vi "GDSLvIcon_AnalyseViIcon.vi"(1 "ViRef/LvCLassRef/LvLibRef/ViPath/2D_Image":variant, 3 "DoATextOCR(False)":bool, 5 "error in (no error)":errorcluster) -> (6 "BodyTextColor":u32(colorbox), 8 "HeaderTextColor":u32(colorbox), 9 "BodyText(OCR)":string, 10 "FrameColor":u32(colorbox), 11 "HeadText(OCR)":string, 12 "FrameThickness(1)":u32=1, 13 "ValidHeaderIcon":bool, 14 "DefaultIcon":bool, 15 "HeaderIcon":u8[][](array[numeric]) format="%x", 16 "HeaderBkColor":u32(colorbox), 17 "BodyIcon":u8[][](array[numeric]) format="%x", 18 "BodyBkColor":u32(colorbox), 19 "error out":errorcluster)   [LabVIEW 2014]
uses:
  <vilib>/picture/picture.llb/imagedata.ctl
  <vilib>/Analysis/NI_AALBase.lvlib
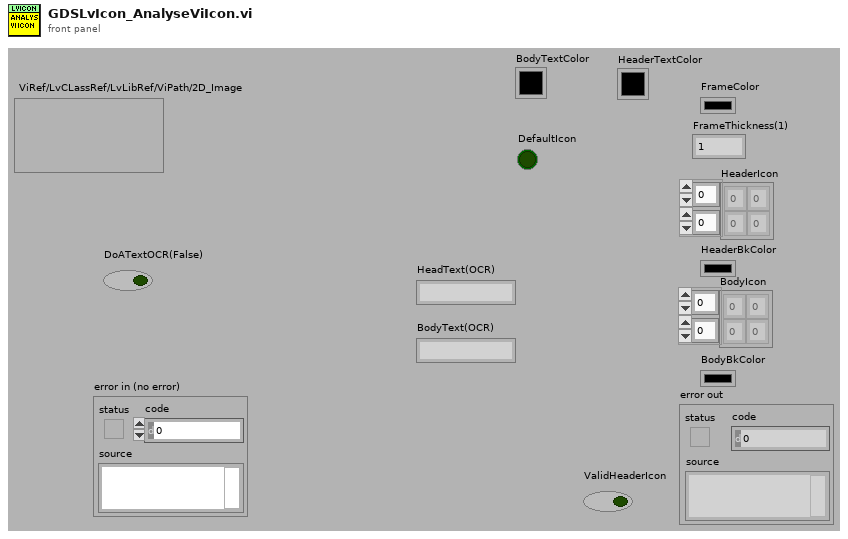
[diagram p1: front panel]
types:
  T1 = cluster{"image":u8[][], "FrameThickness":i32, "FrameColor":u32, "HeaderBkColor":u32, "BodyBkColor":u32, "SplitterAtRow":i32, "Header":u8[][], "Body":u8[][], "HeadTextColor":u32, "BodyTextColor":u32, "BodyBack(8bit)":u8, "BodyText(OCR)":string, "HeadText(OCR)":string, "HeaderBack(8bit)":u8, "EndRow":i32, "StartRow":i32, "BodyTextColor(8bit)":u8, "HeaderTextColor(8bit)":u8, "ShouldHaveHeader":bool}
  T2 = typedef "imagedata.ctl" = cluster{"image type":i32, "image depth":i32, "image":u8[], "mask":u8[], "colors":u32[], "Rectangle":cluster{"left":i16, "top":i16, "right":i16, "bottom":i16}}
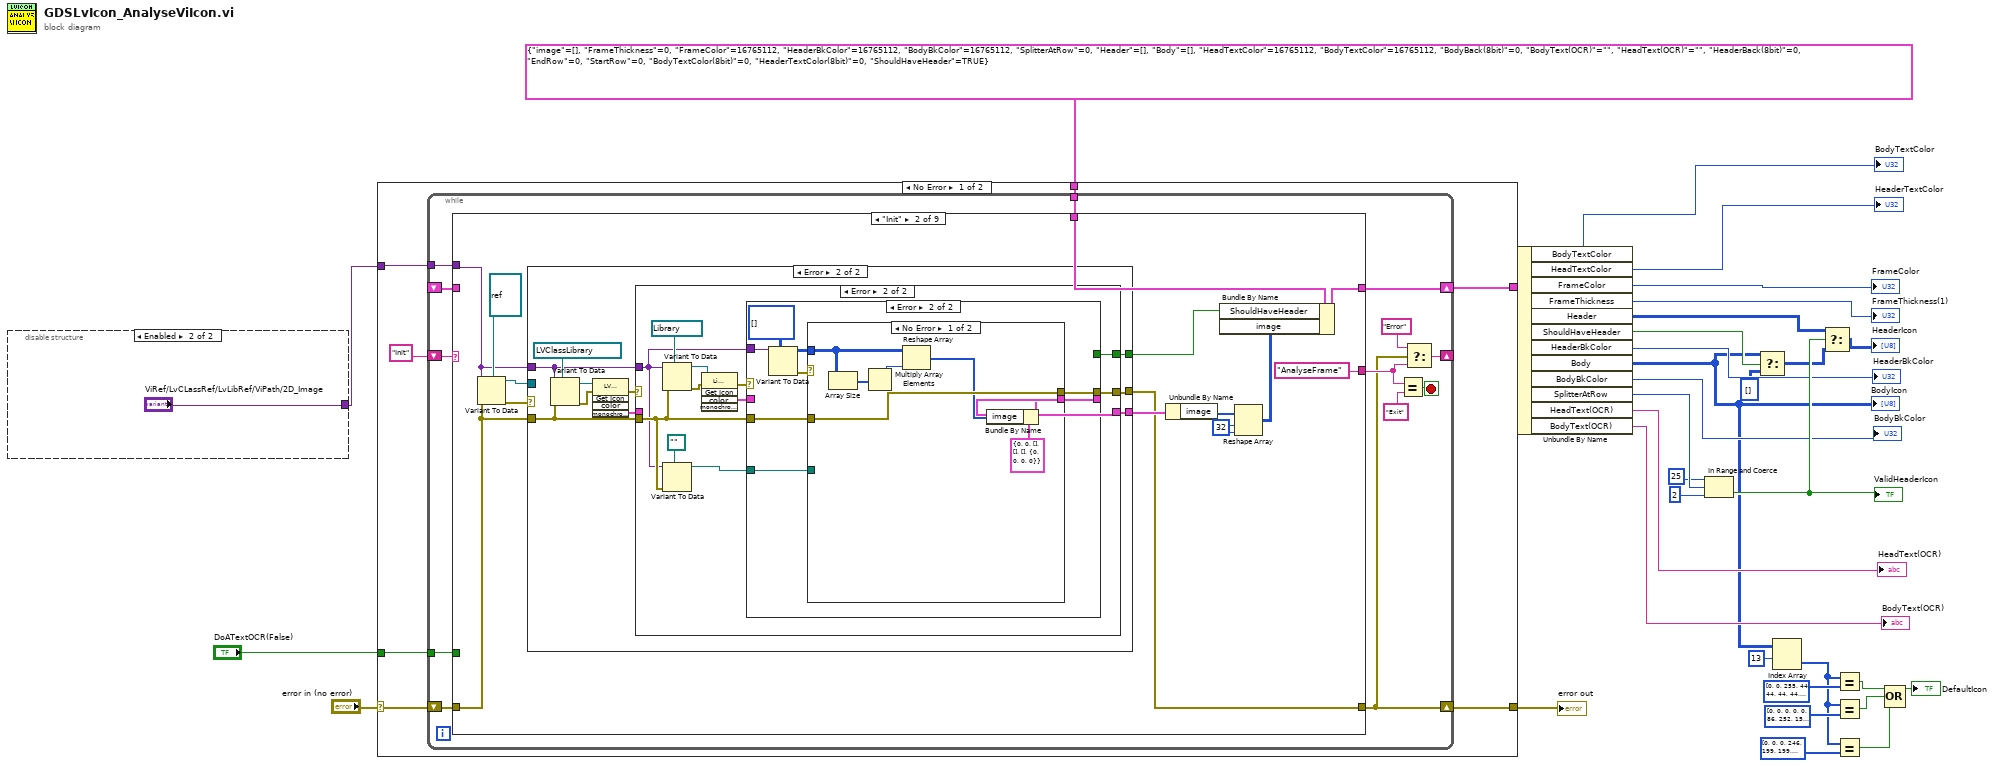
[diagram p0: block diagram]
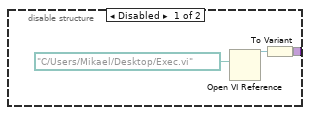
[diagram p2: hidden frame]
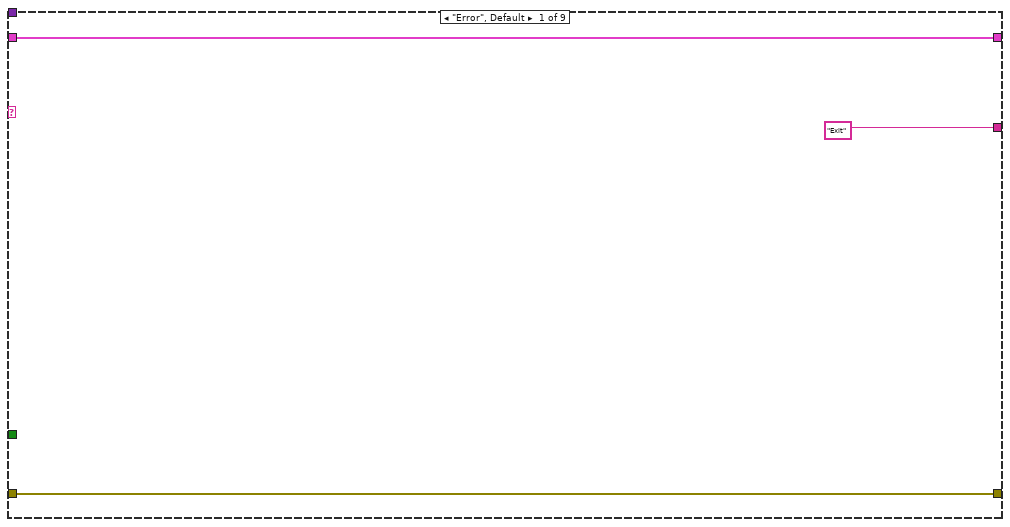
[diagram p3: hidden frame]
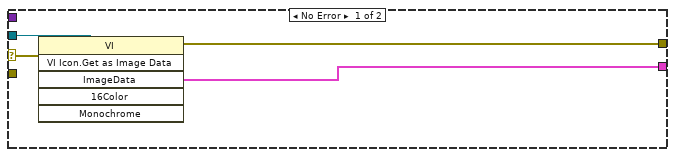
[diagram p4: hidden frame]
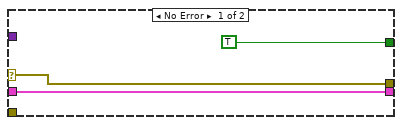
[diagram p6: hidden frame]
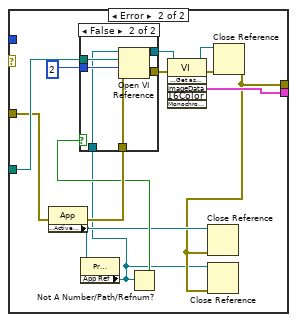
[diagram p7: hidden frame]
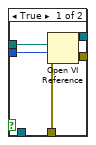
[diagram p8: hidden frame]
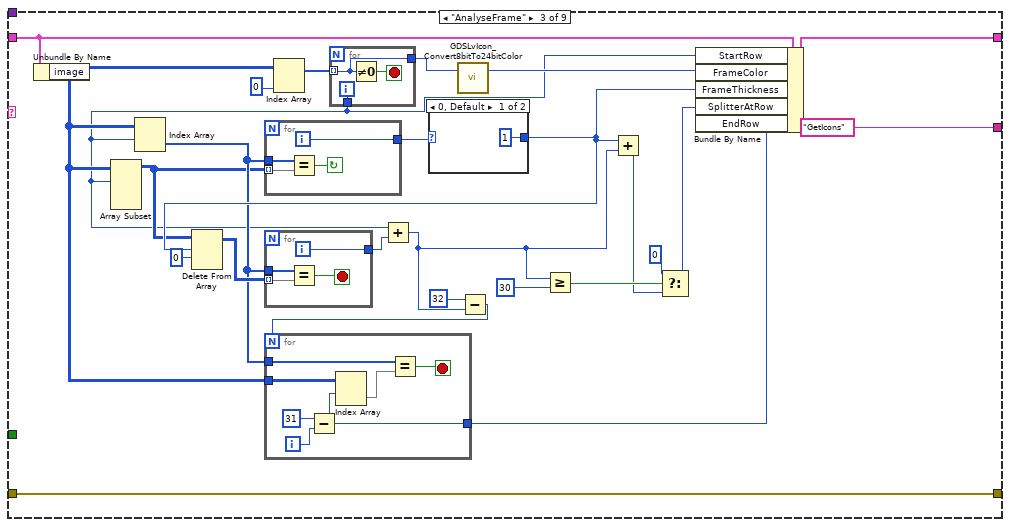
[diagram p9: hidden frame]
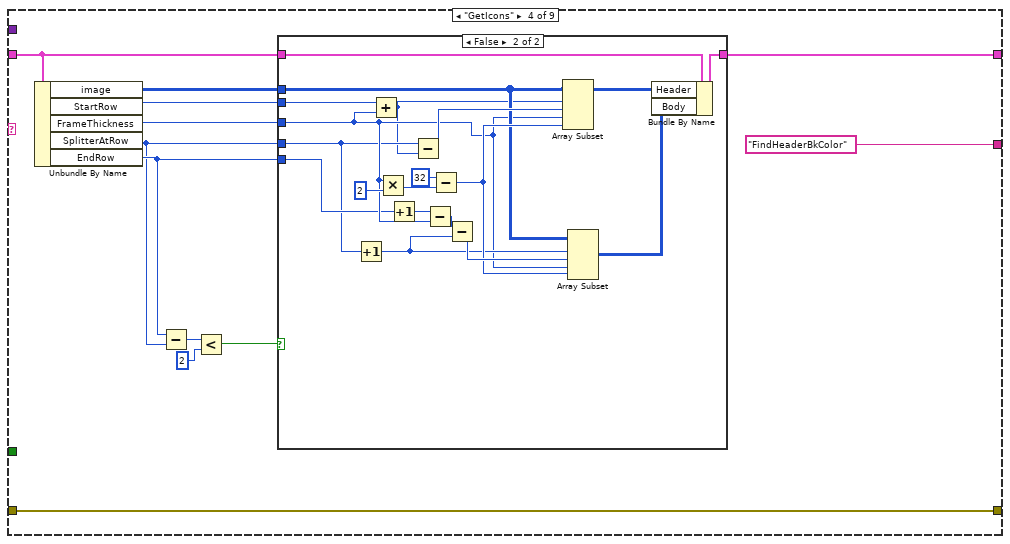
[diagram p11: hidden frame]
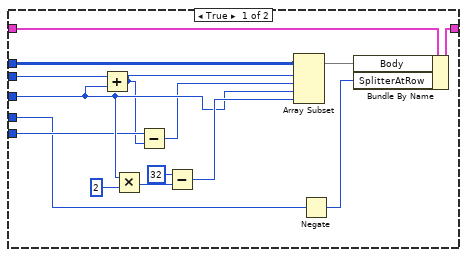
[diagram p12: hidden frame]
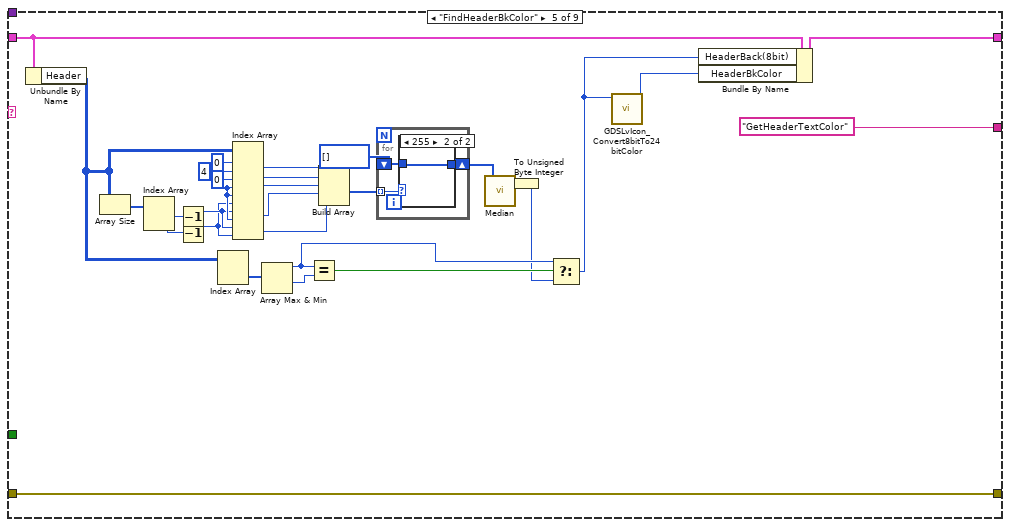
[diagram p13: hidden frame]
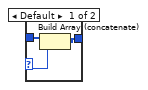
[diagram p14: hidden frame]
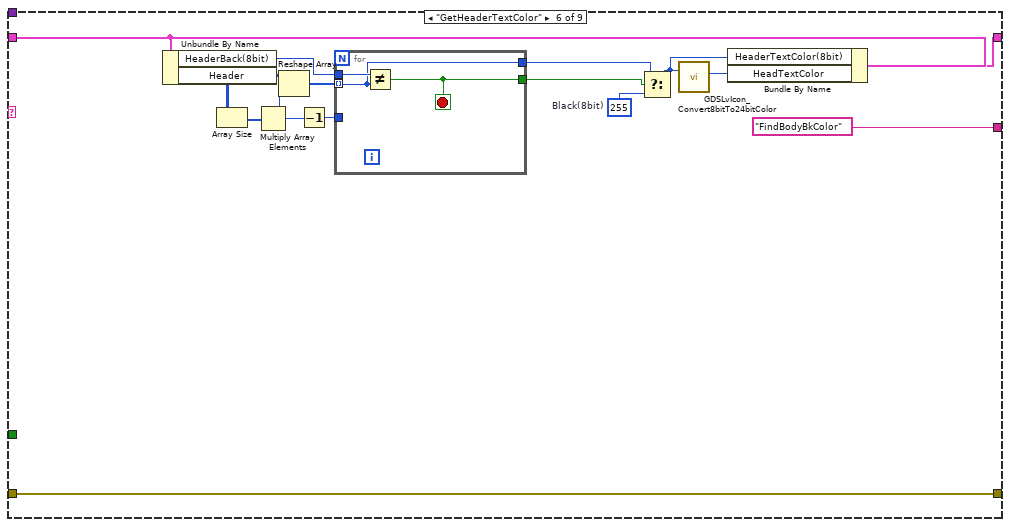
[diagram p15: hidden frame]
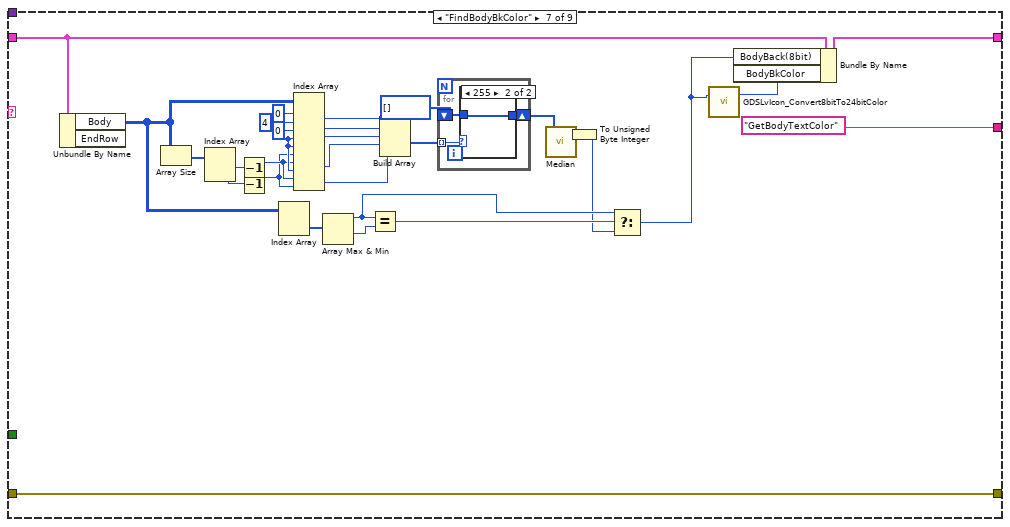
[diagram p16: hidden frame]
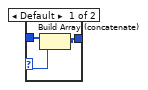
[diagram p17: hidden frame]
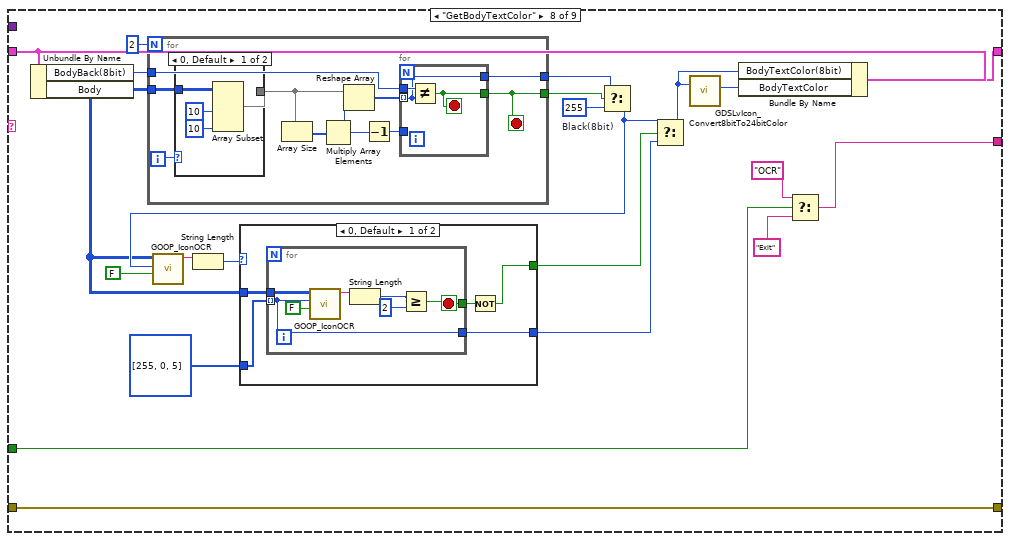
[diagram p18: hidden frame]
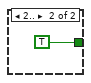
[diagram p19: hidden frame]
diagram:
  n1 = disable-structure shown="Enabled" {
    disable-tunnel: [w34 "ViRef/LvCLassRef/LvLibRef/ViPath/2D_Image"] -> w14
    frame Disabled {
      n2 = Open VI Reference(vi path=path "C:/Users/Mikael/Desktop/Exec.vi") -> (vi reference=w36:refnum<vi>)  [unwired: 5 in, 1 out]
      n3 = To Variant(anything=w36) -> (Variant=w34:variant)
    }
    frame Enabled {
    }
  }
  n4 = case shown="No Error" "error in (no error)" {
    selector: "error in (no error)" -> [w43 w405]
    tunnel: w14 -> [w41 _]
    tunnel: [w42 w405] -> w32
    tunnel: [w40 _] -> w31
    tunnel: T1 {"image"=[], "FrameThickness"=0, "FrameColor"=16765112, "HeaderBkColor"=16765112, "BodyBkColor"=16765112, "SplitterAtRow"=0, "Header"=[], "Body"=[], "HeadTextColor"=16765112, "BodyTextColor"=16765112, "BodyBack(8bit)"=0, "BodyText(OCR)"="", "HeadText(OCR)"="", "HeaderBack(8bit)"=0, "EndRow"=0, "StartRow"=0, "BodyTextColor(8bit)"=0, "HeaderTextColor(8bit)"=0, "ShouldHaveHeader"=TRUE} -> [w39 _]
    tunnel: "DoATextOCR(False)" -> [w38 _]
    frame No Error {
      n5 = while {
        shift-right: [w50] -> w42
        shift-left: w43 -> [w57]
        shift-right: [w55] -> _
        shift-left: "Init" -> [w56]
        shift-right: [w49] -> w40
        shift-left: _ -> [w48]
        tunnel: w41 -> [w47]
        tunnel: w39 -> [w46]
        tunnel: w38 -> [w45]
        stop <- w54 stop-if-true
        n6 = case shown="\"Init\"" w56 {
          tunnel: w57 -> [w60 w64 w165 w199 w264 w286 w319 w348 w389]
          tunnel: [w60 w63 w165 w199 w264 w286 w319 w348 w389] -> w50
          tunnel: ["Exit" "AnalyseFrame" "GetIcons" "FindHeaderBkColor" "GetHeaderTextColor" "FindBodyBkColor" "GetBodyTextColor" w339 "Exit"] -> w51
          tunnel: [w58 w72 w169 w201 w262 w284 w317 w346 w394] -> w49
          tunnel: w48 -> [w58 _ w170 w202 w263 w285 w318 w347 w392]
          tunnel: w47 -> [_ w67 _ _ _ _ _ _ _]
          tunnel: w46 -> [_ w70 _ _ _ _ _ _ _]
          tunnel: w45 -> [_ _ _ _ _ _ _ w341 _]
          frame "Error", Default {
          }
          frame "Init" {
            w61 = 32 ("dimension size")
            n7 = Variant To Data(error in=w64, type=refnum<vi> refnum ("ViRef or LvCLassRef"), Variant=w67) -> (data=w66:refnum<vi>, error out=w68:errorcluster)
            n8 = case shown="Error" w68 {
              selector: w68 -> [w77 _]
              tunnel: w67 -> [_ w81]
              tunnel: w66 -> [w78 _]
              tunnel: [w76 w82] -> w65
              tunnel: w64 -> [_ w80]
              tunnel: [w75 w84] -> w63
              tunnel: [_ w79] -> w62
              frame No Error {
                n9 = invoke class="VI" method="VI Icon.Get as Image Data"(reference=w78, error in=w77) -> (error out=w75:errorcluster, "ImageData"=w76:T2)  [unwired: 4 in, 4 out]
              }
              frame Error {
                n10 = Variant To Data(error in=w80, type=refnum<vi> refnum ("LVClassLibrary Refnum"), Variant=w81) -> (data=w87:refnum<vi>, error out=w86:errorcluster)
                n11 = invoke class="LVClassLibrary" method="Get Icon"(reference=w87, error in=w86) -> (error out=w85:errorcluster, "color"=w83:T2)  [unwired: 3 in, 3 out]
                n12 = case shown="Error" w85 {
                  selector: w85 -> [w90 _]
                  tunnel: [w90 w96] -> w84
                  tunnel: w83 -> [w89 _]
                  tunnel: [w89 w97] -> w82
                  tunnel: w81 -> [_ w91]
                  tunnel: w80 -> [_ w93]
                  tunnel: [_ w92] -> w79
                  frame No Error {
                  }
                  frame Error {
                    n13 = Variant To Data(error in=w93, type=refnum<vi> refnum ("Library Refnum"), Variant=w91) -> (data=w101:refnum<vi>, error out=w100:errorcluster)
                    n14 = Variant To Data(error in=w93, type=path "", Variant=w91) -> (data=w94:path)  [unwired: 1 out]
                    n15 = invoke class="Library" method="Get Icon"(reference=w101, error in=w100) -> (error out=w99:errorcluster, "color"=w98:T2)  [unwired: 3 in, 3 out]
                    n16 = case shown="Error" w99 {
                      selector: w99 -> [w104 _]
                      tunnel: w98 -> [w105 _]
                      tunnel: [w105 w112] -> w97
                      tunnel: [w104 w110] -> w96
                      tunnel: w94 -> [_ w113]
                      tunnel: w93 -> [_ w111]
                      tunnel: [TRUE _] -> w92
                      tunnel: w91 -> [_ w109]
                      frame No Error {
                      }
                      frame Error {
                        n17 = Variant To Data(type=u8[][] [] ("output array"), Variant=w109) -> (data=w106:u8[][], error out=w107:errorcluster)  [unwired: 1 in]
                        n18 = case shown="No Error" w107 {
                          tunnel: w113 -> [_ w133]
                          tunnel: [w118 w128] -> w112
                          tunnel: w111 -> [w120 w126]
                          tunnel: [w120 w122] -> w110
                          tunnel: w106 -> [w117 _]
                          frame No Error {
                            n19 = Array Size(array=w117) -> (size(s)=w115:i32[])
                            n20 = Multiply Array Elements(1:w115) -> (0:w116:i32)
                            n21 = Reshape Array(w117, w116) -> (w114:u8[])
                            n22 = Bundle By Name(cluster=T2 {"image type"=0, "image depth"=0, "image"=[], "mask"=[], "colors"=[], "Rectangle"={"left"=0, "top"=0, "right"=0, "bottom"=0}} ("ImageData"), "image"=w114) -> (w118:T2)
                          }
                          frame Error {
                            n23 = property class="App"(error in=w126) -> (error out=w125:errorcluster, "Project:Active Project"=w123:refnum<vi>)  [unwired: 1 in, 1 out]
                            n24 = property class="Project"(reference=w123) -> ("App Ref"=w121:refnum<vi>)  [unwired: 1 in, 2 out]
                            n25 = Not A Number/Path/Refnum?(number/path/refnum=w121) -> (NaN/Path/Refnum?=w124:bool)
                            n26 = case shown="False" w124 {
                              tunnel: w133 -> [w138 w144]
                              tunnel: [w137 w143] -> w132
                              tunnel: [w136 w142] -> w131
                              tunnel: 2 ("options") -> [w135 w141]
                              tunnel: w125 -> [w134 w140]
                              tunnel: w121 -> [_ w139]
                              frame True {
                                n27 = Open VI Reference(vi path=w138, options=w135, error in (no error)=w134) -> (vi reference=w136:refnum<vi>, error out=w137:errorcluster)  [unwired: 3 in]
                              }
                              frame False {
                                n28 = Open VI Reference(application reference (local)=w139, vi path=w144, options=w141, error in (no error)=w140) -> (vi reference=w142:refnum<vi>, error out=w143:errorcluster)  [unwired: 2 in]
                              }
                            }
                            n29 = invoke class="VI" method="VI Icon.Get as Image Data"(reference=w131, error in=w132) -> (reference out=w129:refnum<vi>, error out=w130:errorcluster, "ImageData"=w128:T2)  [unwired: 4 in, 3 out]
                            n30 = Close Reference(reference=w129, error in (no error)=w130) -> (error out=w122:errorcluster)
                            n31 = Close Reference(reference=w123, error in (no error)=w122) -> ()  [unwired: 1 out]
                            n32 = Close Reference(reference=w121, error in (no error)=w122) -> ()  [unwired: 1 out]
                          }
                        }
                      }
                    }
                  }
                }
              }
            }
            n33 = Unbundle By Name(w65) -> ("image"=w73:u8[])
            n34 = Reshape Array(w73, w61, w61) -> (w71:u8[][])
            n35 = Bundle By Name(cluster=w70, "ShouldHaveHeader"=w62, "image"=w71) -> (w72:T1)
          }
          frame "AnalyseFrame" {
            n36 = Unbundle By Name(w170) -> ("image"=w149:u8[][])
            n37 = Index Array(array=w149, index (col)=0 ("index (row)")) -> (element=w154:u8[])  [unwired: 1 in]
            n38 = for {
              tunnel: w154 -> [w172] mode=indexing
              tunnel: [w172] -> w153
              tunnel: [w171] -> w147
              i -> [w171]
              stop <- w173 stop-if-true
              n39 = Not Equal To 0?(x=w172) -> (x != 0?=w173:bool)
            }
            n40 = Array Subset(array=w149, index (row)=w147) -> (w151:u8[][])  [unwired: 3 in]
            n41 = Index Array(array=w149, index (row)=w147) -> (element=w157:u8[])  [unwired: 1 in]
            n42 = for {
              tunnel: w151 -> [w188] mode=indexing
              tunnel: w157 -> [w187]
              tunnel: [w186] -> w164
              i -> [w186]
              stop <- w185 continue-if-true
              n43 = Equal?(x=w187, y=w188) -> (x = y?=w185:bool)
            }
            n44 = case shown="0, Default" w164 {
              selector: w164 -> [_ w190]
              tunnel: [1 w190] -> w163
              frame 0, Default {
              }
              frame 1..3 {
              }
            }
            n45 = Delete From Array(array=w151, length=w163, index (row)=0) -> (array with subset deleted=w167:u8[][])  [unwired: 1 in, 1 out]
            n46 = for {
              tunnel: w167 -> [w182] mode=indexing
              tunnel: w157 -> [w184]
              tunnel: [w183] -> w145
              i -> [w183]
              stop <- w181 stop-if-true
              n47 = Equal?(x=w184, y=w182) -> (x = y?=w181:bool)
            }
            n48 = Add(x=w147, y=w145) -> (x+y=w146:i32)
            n49 = call <resource>:"GDSLvIcon_Convert8bitTo24bitColor.vi"("Color8bit"=w153) -> ("Color24bit"=w158:u32)  [unwired: 17 in, 1 out]
            n50 = Subtract(x=32 ("y"), y=w146) -> (x-y=w155:i32)
            n51 = for {
              N: w155 -> [_]
              tunnel: w157 -> [w180]
              tunnel: w149 -> [w176]
              tunnel: [w174] -> w148
              i -> [w177]
              stop <- w179 stop-if-true
              n52 = Subtract(x=31 ("y"), y=w177) -> (x-y=w174:i32)
              n53 = Index Array(array=w176, index (row)=w174) -> (element=w175:u8[])  [unwired: 1 in]
              n54 = Equal?(x=w180, y=w175) -> (x = y?=w179:bool)
            }
            n55 = Greater Or Equal?(x=w146, y=30) -> (x >= y?=w161:bool)
            n56 = Add(x=w163, y=w146) -> (x+y=w150:i32)
            n57 = Select(t=0, s=w161, f=w150) -> (s? t:f=w159:i32)
            n58 = Bundle By Name(cluster=w170, "StartRow"=w147, "FrameColor"=w158, "FrameThickness"=w163, "SplitterAtRow"=w159, "EndRow"=w148) -> (w169:T1)
          }
          frame "GetIcons" {
            n59 = Unbundle By Name(w202) -> ("image"=w198:u8[][], "StartRow"=w196:i32, "FrameThickness"=w197:i32, "SplitterAtRow"=w194:i32, "EndRow"=w195:i32)
            n60 = Subtract(x=w195, y=w194) -> (x-y=w193:i32)
            n61 = Less?(x=w193, y=2) -> (x < y?=w191:bool)
            n62 = case shown="False" w191 {
              tunnel: w202 -> [w217 w236]
              tunnel: [w216 w235] -> w201
              tunnel: w198 -> [w210 w224]
              tunnel: w197 -> [w209 w223]
              tunnel: w196 -> [w208 w222]
              tunnel: w195 -> [w207 w221]
              tunnel: w194 -> [w204 w220]
              frame True {
                n63 = Add(x=w208, y=w209) -> (x+y=w206:i32)
                n64 = Multiply(x=w209, y=2) -> (x*y=w213:i32)
                n65 = Subtract(x=w207, y=w206) -> (x-y=w205:i32)
                n66 = Subtract(x=32, y=w213) -> (x-y=w212:i32)
                n67 = Array Subset(array=w210, index (row)=w206, length (row)=w205, index (col)=w209, length (col)=w212) -> (w215:u8[][])
                n68 = Negate(x=w204) -> (-x=w203:i32)
                n69 = Bundle By Name(cluster=w217, "Body"=w215, "SplitterAtRow"=w203) -> (w216:T1)
              }
              frame False {
                n70 = Increment(x=w220) -> (x+1=w225:i32)
                n71 = Add(x=w222, y=w223) -> (x+y=w219:i32)
                n72 = Multiply(x=w223, y=2) -> (x*y=w231:i32)
                n73 = Increment(x=w221) -> (x+1=w218:i32)
                n74 = Subtract(x=w220, y=w219) -> (x-y=w233:i32)
                n75 = Subtract(x=w218, y=w223) -> (x-y=w226:i32)
                n76 = Subtract(x=32, y=w231) -> (x-y=w229:i32)
                n77 = Subtract(x=w226, y=w225) -> (x-y=w230:i32)
                n78 = Array Subset(array=w224, index (row)=w219, length (row)=w233, index (col)=w223, length (col)=w229) -> (w234:u8[][])
                n79 = Array Subset(array=w224, index (row)=w225, length (row)=w230, index (col)=w223, length (col)=w229) -> (w228:u8[][])
                n80 = Bundle By Name(cluster=w236, "Header"=w234, "Body"=w228) -> (w235:T1)
              }
            }
          }
          frame "FindHeaderBkColor" {
            w257 = 0 ("index (row)")
            n81 = Unbundle By Name(w263) -> ("Header"=w239:u8[][])
            n82 = Array Size(array=w239) -> (size(s)=w260:i32[])
            n83 = Index Array(array=w260) -> (element #1=w259:i32, element #2=w258:i32)  [unwired: 2 in]
            n84 = Decrement(x=w259) -> (x-1=w256:i32)
            n85 = Decrement(x=w258) -> (x-1=w255:i32)
            n86 = Index Array(array=w239) -> (element=w250:u8[])  [unwired: 2 in]
            n87 = Index Array(array=w239, index (row) #1=0 ("index (row)"), index (col) #1=4 ("disabled index (col)"), index (row) #2=w257, index (col) #2=w257, index (row) #3=w257, index (col) #3=w255, index (row) #4=w256, index (col) #4=w257, index (row) #5=w256, index (col) #5=w255) -> (element #1=w243:u8, element #2=w254:u8, element #3=w253:u8, element #4=w252:u8, element #5=w251:u8)
            n88 = Array Max & Min(array=w250) -> (max value=w247:u8, min value=w249:u8)  [unwired: 2 out]
            n89 = Equal?(x=w247, y=w249) -> (x = y?=w248:bool)
            n90 = Build Array(w243, w254, w253, w252, w251) -> (w242:u8[])
            n91 = for {
              tunnel: w242 -> [w268] mode=indexing
              shift-right: [w266] -> w240
              shift-left: u8[] [] -> [w267]
              n92 = case shown="255" w268 {
                selector: w268 -> [w269 _]
                tunnel: w267 -> [w271 w272]
                tunnel: [w270 w272] -> w266
                frame Default {
                  n93 = Build Array (concatenate)(w271, w269) -> (w270:u8[])
                }
                frame 255 {
                }
              }
            }
            n94 = call <vilib>:"Median.vi"("X"=w240) -> ("median"=w246:dbl)  [unwired: 1 out]
            n95 = To Unsigned Byte Integer(number=w246) -> (unsigned 8bit integer=w237:u8)
            n96 = Select(t=w247, s=w248, f=w237) -> (s? t:f=w238:u8)
            n97 = call <resource>:"GDSLvIcon_Convert8bitTo24bitColor.vi"("Color8bit"=w238) -> ("Color24bit"=w261:u32)  [unwired: 17 in, 1 out]
            n98 = Bundle By Name(cluster=w263, "HeaderBack(8bit)"=w238, "HeaderBkColor"=w261) -> (w262:T1)
          }
          frame "GetHeaderTextColor" {
            w274 = u8 255  # Black(8bit)
            n99 = Unbundle By Name(w285) -> ("HeaderBack(8bit)"=w279:u8, "Header"=w282:u8[][])
            n100 = Array Size(array=w282) -> (size(s)=w281:i32[])
            n101 = Multiply Array Elements(1:w281) -> (0:w278:i32)
            n102 = Reshape Array(w282, w278) -> (w280:u8[])
            n103 = Decrement(x=w278) -> (x-1=w277:i32)
            n104 = for {
              tunnel: w280 -> [w289] mode=indexing
              tunnel: w279 -> [w290]
              tunnel: w277 -> [_]
              tunnel: [w288] -> w276
              tunnel: [w289] -> w275
              stop <- w288 stop-if-true
              n105 = Not Equal?(x=w290, y=w289) -> (x != y?=w288:bool)
            }
            n106 = Select(t=w275, s=w276, f=w274) -> (s? t:f=w273:u8)
            n107 = call <resource>:"GDSLvIcon_Convert8bitTo24bitColor.vi"("Color8bit"=w273) -> ("Color24bit"=w283:u32)  [unwired: 17 in, 1 out]
            n108 = Bundle By Name(cluster=w285, "HeaderTextColor(8bit)"=w273, "HeadTextColor"=w283) -> (w284:T1)
          }
          frame "FindBodyBkColor" {
            w313 = 0 ("index (row)")
            n109 = Unbundle By Name(w318) -> ("Body"=w304:u8[][])  [unwired: 1 out]
            n110 = Array Size(array=w304) -> (size(s)=w316:i32[])
            n111 = Index Array(array=w316) -> (element #1=w315:i32, element #2=w314:i32)  [unwired: 2 in]
            n112 = Decrement(x=w315) -> (x-1=w312:i32)
            n113 = Decrement(x=w314) -> (x-1=w311:i32)
            n114 = Index Array(array=w304) -> (element=w303:u8[])  [unwired: 2 in]
            n115 = Index Array(array=w304, index (row) #1=0 ("index (row)"), index (col) #1=4 ("disabled index (col)"), index (row) #2=w313, index (col) #2=w313, index (row) #3=w313, index (col) #3=w311, index (row) #4=w312, index (col) #4=w313, index (row) #5=w312, index (col) #5=w311) -> (element #1=w295:u8, element #2=w310:u8, element #3=w309:u8, element #4=w308:u8, element #5=w307:u8)
            n116 = Array Max & Min(array=w303) -> (max value=w300:u8, min value=w302:u8)  [unwired: 2 out]
            n117 = Equal?(x=w300, y=w302) -> (x = y?=w301:bool)
            n118 = Build Array(w295, w310, w309, w308, w307) -> (w294:u8[])
            n119 = for {
              tunnel: w294 -> [w322] mode=indexing
              shift-right: [w320] -> w292
              shift-left: u8[] [] -> [w321]
              n120 = case shown="255" w322 {
                selector: w322 -> [w323 _]
                tunnel: w321 -> [w325 w326]
                tunnel: [w324 w326] -> w320
                frame Default {
                  n121 = Build Array (concatenate)(w325, w323) -> (w324:u8[])
                }
                frame 255 {
                }
              }
            }
            n122 = call <vilib>:"Median.vi"("X"=w292) -> ("median"=w299:dbl)  [unwired: 1 out]
            n123 = To Unsigned Byte Integer(number=w299) -> (unsigned 8bit integer=w291:u8)
            n124 = Select(t=w300, s=w301, f=w291) -> (s? t:f=w298:u8)
            n125 = call <resource>:"GDSLvIcon_Convert8bitTo24bitColor.vi"("Color8bit"=w298) -> ("Color24bit"=w306:u32)  [unwired: 17 in, 1 out]
            n126 = Bundle By Name(cluster=w318, "BodyBack(8bit)"=w298, "BodyBkColor"=w306) -> (w317:T1)
          }
          frame "GetBodyTextColor" {
            w337 = u8 255  # Black(8bit)
            n127 = Unbundle By Name(w347) -> ("BodyBack(8bit)"=w344:u8, "Body"=w330:u8[][])
            n128 = for {
              N: 2 -> [_]
              tunnel: w330 -> [w365]
              tunnel: w344 -> [w369]
              tunnel: [w362] -> w343
              tunnel: [w366] -> w342
              i -> [w363]
              stop <- w362 stop-if-true
              n129 = case shown="0, Default" w363 {
                tunnel: w365 -> [w375 w376]
                tunnel: [w374 w376] -> w364
                frame 0, Default {
                  n130 = Array Subset(array=w375, length (row)=10 ("length"), length (col)=10 ("length")) -> (w374:u8[][])  [unwired: 2 in]
                }
                frame 1 {
                }
              }
              n131 = Array Size(array=w364) -> (size(s)=w371:i32[])
              n132 = Multiply Array Elements(1:w371) -> (0:w368:i32)
              n133 = Reshape Array(w364, w368) -> (w370:u8[])
              n134 = Decrement(x=w368) -> (x-1=w367:i32)
              n135 = for {
                tunnel: w370 -> [w378] mode=indexing
                tunnel: w369 -> [w379]
                tunnel: w367 -> [_]
                tunnel: [w377] -> w362
                tunnel: [w378] -> w366
                stop <- w377 stop-if-true
                n136 = Not Equal?(x=w379, y=w378) -> (x != y?=w377:bool)
              }
            }
            n137 = Select(t=w342, s=w343, f=w337) -> (s? t:f=w334:u8)
            n138 = call <resource>:"GOOP_IconOCR.vi"("BackColor(T), TextColor(F)"=FALSE, "BackColor Or TextColor(8bit)"=w334, "Icon"=w330) -> ("String"=w332:string)  [unwired: 8 in]
            n139 = String Length(string=w332) -> (length=w331:i32)
            n140 = case shown="0, Default" w331 {
              tunnel: w330 -> [w353 _]
              tunnel: u8[] [255, 0, 5] -> [w352 _]
              tunnel: [w350 TRUE] -> w328
              tunnel: [w349 _] -> w327
              frame 0, Default {
                n141 = for {
                  tunnel: w353 -> [w358]
                  tunnel: w352 -> [w354] mode=indexing
                  tunnel: [w355] -> w351
                  tunnel: [w354] -> w349
                  stop <- w355 stop-if-true
                  n142 = call <resource>:"GOOP_IconOCR.vi"("BackColor(T), TextColor(F)"=FALSE, "BackColor Or TextColor(8bit)"=w354, "Icon"=w358) -> ("String"=w360:string)  [unwired: 8 in]
                  n143 = String Length(string=w360) -> (length=w357:i32)
                  n144 = Greater Or Equal?(x=w357, y=2) -> (x >= y?=w355:bool)
                }
                n145 = Not(x=w351) -> (.not. x?=w350:bool)
              }
              frame 2.. {
              }
            }
            n146 = Select(t=w334, s=w328, f=w327) -> (s? t:f=w335:u8)
            n147 = call <resource>:"GDSLvIcon_Convert8bitTo24bitColor.vi"("Color8bit"=w335) -> ("Color24bit"=w345:u32)  [unwired: 17 in, 1 out]
            n148 = Bundle By Name(cluster=w347, "BodyTextColor(8bit)"=w335, "BodyTextColor"=w345) -> (w346:T1)
            n149 = Select(t="OCR", s=w341, f="Exit") -> (s? t:f=w339:string)
          }
          frame "OCR" {
            w381 = bool[] [FALSE, TRUE]
            n150 = Unbundle By Name(w392) -> ("Header"=w385:u8[][], "HeaderTextColor(8bit)"=w383:u8, "HeaderBack(8bit)"=w382:u8)  [unwired: 1 out]
            n151 = Unbundle By Name(w392) -> ("Body"=w390:u8[][], "BodyTextColor(8bit)"=w386:u8, "BodyBack(8bit)"=w387:u8)
            n152 = Build Array(w386, w387) -> (w388:u8[])
            n153 = Build Array(w383, w382) -> (w384:u8[])
            n154 = for {
              tunnel: [w402] -> w391
              tunnel: w390 -> [w404]
              tunnel: w381 -> [w403] mode=indexing
              tunnel: w388 -> [w400] mode=indexing
              stop <- w401 continue-if-true
              n155 = call <resource>:"GOOP_IconOCR.vi"("BackColor(T), TextColor(F)"=w403, "BackColor Or TextColor(8bit)"=w400, "Icon"=w404) -> ("String"=w402:string)  [unwired: 8 in]
              n156 = Empty String/Path?(string/path=w402) -> (empty?=w401:bool)
            }
            n157 = for {
              tunnel: [w397] -> w380
              tunnel: w385 -> [w399]
              tunnel: w381 -> [w398] mode=indexing
              tunnel: w384 -> [w395] mode=indexing
              stop <- w396 continue-if-true
              n158 = call <resource>:"GOOP_IconOCR.vi"("BackColor(T), TextColor(F)"=w398, "BackColor Or TextColor(8bit)"=w395, "Icon"=w399) -> ("String"=w397:string)  [unwired: 8 in]
              n159 = Empty String/Path?(string/path=w397) -> (empty?=w396:bool)
            }
            n160 = Bundle By Name(cluster=w392, "BodyText(OCR)"=w391, "HeadText(OCR)"=w380) -> (w394:T1)
          }
        }
        n161 = Equal?(x=w51, y="Exit") -> (x = y?=w54:bool)
        n162 = Select(t="Error", s=w50, f=w51) -> (s? t:f=w55:string)
      }
    }
    frame Error {
    }
  }
  "error out" <- w32
  n163 = Unbundle By Name(w31) -> ("BodyTextColor"=→"BodyTextColor":u32, "HeadTextColor"=→"HeaderTextColor":u32, "FrameColor"=→"FrameColor":u32, "FrameThickness"=→"FrameThickness(1)":i32, "Header"=w24:u8[][], "ShouldHaveHeader"=w13:bool, "HeaderBkColor"=→"HeaderBkColor":u32, "Body"=w5:u8[][], "BodyBkColor"=→"BodyBkColor":u32, "SplitterAtRow"=w28:i32, "HeadText(OCR)"=→"HeadText(OCR)":string, "BodyText(OCR)"=→"BodyText(OCR)":string)
  "BodyIcon" <- w5
  n164 = In Range and Coerce(upper limit=25 ("x"), x=w28, lower limit=2) -> (In Range?=w22:bool)  [unwired: 1 out]
  "ValidHeaderIcon" <- w22
  n165 = Select(t=w5, s=w13, f=u8[][] []) -> (s? t:f=w11:u8[][])
  n166 = Index Array(array=w5, index (row)=13) -> (element=w3:u8[])  [unwired: 1 in]
  n167 = Select(t=w24, s=w22, f=w11) -> (s? t:f=→"HeaderIcon":u8[][])
  n168 = Equal?(x=w3, y=u8[] [0, 0, 255, 44, 44, 44, 44, 44, 44, 44, 44, 44, 44, 44, 44, 44, 44, 44, 131, 5, 131, 131, 0, 0, 0, 0, 0, 0, 0, 0] ("subarray")) -> (x = y?=w9:bool)
  n169 = Equal?(x=w3, y=u8[] [0, 0, 0, 0, 0, 86, 252, 153, 74, 117, 116, 117, 172, 43, 0, 0, 0, 0, 0, 0, 0, 0, 0, 0, 0, 0, 0, 0, 0, 0] ("subarray 2")) -> (x = y?=w6:bool)
  n170 = Equal?(x=w3, y=u8[] [0, 0, 0, 246, 199, 199, 206, 199, 200, 202, 230, 203, 200, 199, 199, 206, 165, 165, 165, 43, 0, 0, 0, 0, 0, 0, 0, 0, 0, 0] ("subarray")) -> (x = y?=w1:bool)
  n171 = Compound Arithmetic op=OR(w9, w6, w1) -> (→"DefaultIcon":bool)
